vi "Construct Handle Mouse Down Msg.vi"(7 "Return Priority (Normal)":T1=enum."Normal", 11 "Return Enqueuer":refnum<class "Message Enqueuer.lvclass">) -> (3 "Handle Mouse Down Msg out":refnum<class "Handle Mouse Down Msg.lvclass">)   [LabVIEW 2017, in "Handle Mouse Down Msg.lvclass"]
uses:
  Handle Mouse Down Msg.lvclass
  <vilib>/gpm_packages/@cs/actor-framework-messages/Source/RoundTripMessage/RoundTripMessage.lvclass
  C:/Users/jonmc/Documents/Git/Test Executive Builder/gpm_packages/@cs/actor-framework-messages/Source/RoundTripMessage/RoundTripMessage.lvclass
  <vilib>/ActorFramework/Message Enqueuer/Message Enqueuer.lvclass
  <vilib>/ActorFramework/Message Enqueuer/Message Priority.ctl
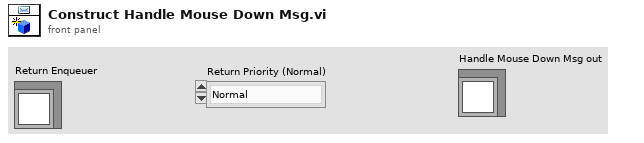
[diagram p1: front panel]
types:
  T1 = typedef "Actor Framework.lvlib/Message Enqueuer.lvclass/Message Priority.ctl" = enum16{"Low", "Normal", "High"}
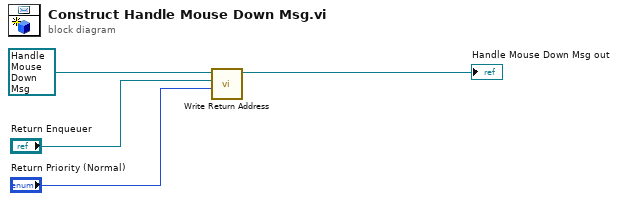
[diagram p0: block diagram]
diagram:
  n1 = call <vilib>:"Write Return Address.vi"("Return Priority (Normal)"="Return Priority (Normal)", "Return Enqueuer"="Return Enqueuer", "RoundTripMessage In"=refnum<class "Handle Mouse Down Msg.lvclass"> refnum ("Handle Mouse Down Msg in")) -> ("RoundTripMessage Out"=→"Handle Mouse Down Msg out":refnum<class "Handle Mouse Down Msg.lvclass">)  [unwired: 8 in]
